vi "DIALOG_Single Element Cluster.vi"(10 "Display Items":T2[](array[typedef]), 11 "Affected Items":T1) -> (2 "Placement Out":enum32{"Choice 1", "Choice 2"}(radio), 3 "Selected Items (tags)":string[](array[string]))   [LabVIEW 2023]
uses:
  cluster/Cluster Element Description.ctl
  top/BundleMagic.ctl
panel:
  out "Cancel?":bool
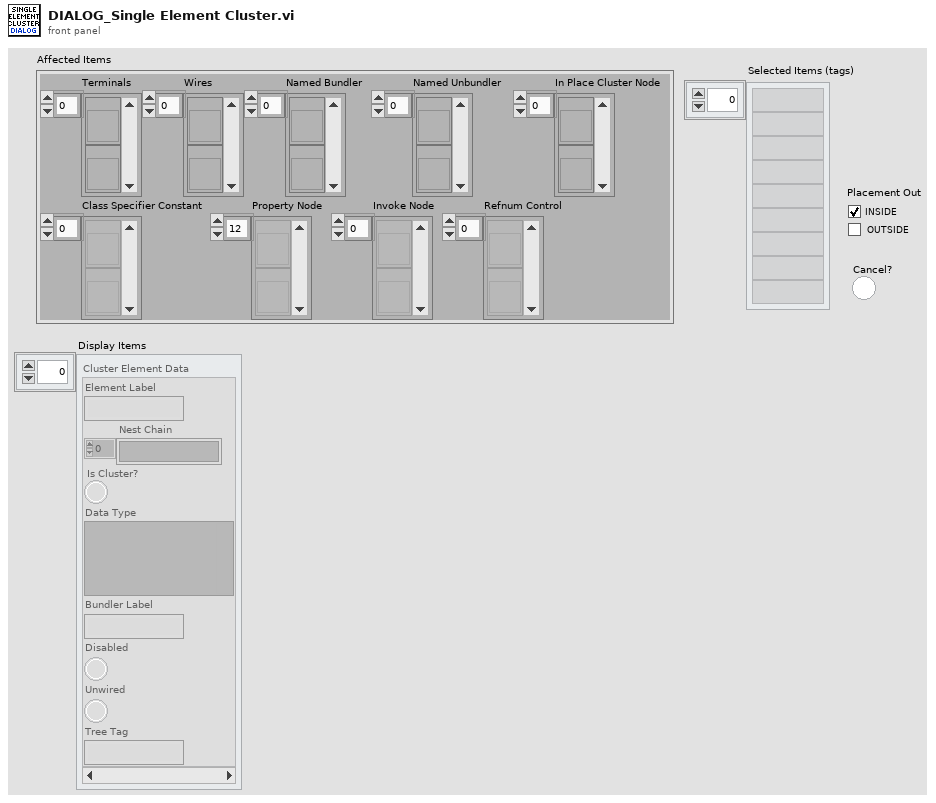
[diagram p1: front panel]
types:
  T1 = typedef "BundleMagic.ctl" = cluster{"Terminals":refnum<vi>[], "Wires":refnum<vi>[], "Named Bundler":refnum<vi>[], "Named Unbundler":refnum<vi>[], "In Place Cluster Node":refnum<vi>[], "Class Specifier Constant":refnum<vi>[], "Property Node":refnum<vi>[], "Invoke Node":refnum<vi>[], "Refnum Control":refnum<vi>[]}
  T2 = typedef "Cluster Element Description.ctl" = cluster{"Element Label":string, "Nest Chain":string[], "Is Cluster?":bool, "Data Type":variant, "Bundler Label":string, "Disabled":bool, "Unwired":bool, "Tree Tag":string}
  T3 = cluster{"Tunnel Ref":refnum<vi>, "On Tunnel?":bool, "Placement":enum32{"Choice 1", "Choice 2"}, "Tunnel Is Indexing?":bool, "Diagram":refnum<vi>, "Position":cluster{"Refnum":refnum<vi>, "Relative Direction":enum32{"Right", "Left", "Top", "Bottom", "Top Right", "Top Left", "Bottom Right", "Bottom Left"}, "Point32":cluster{"Horizontal":i32, "Vertical":i32}}, "Chosen Terminal":refnum<vi>, "Is Refnum?":bool, "Is Cluster?":bool, "Is Source?":bool, "Tunnel Direction":enum16{"In-Going", "Out-Going"}, "Tunnel Position":enum16{"Left", "Top", "Right", "Bottom"}, "Is Inner?":bool, "Terminal Is Indexing?":bool}
  T4 = enum16{"Left Button", "Center Button", "Right Button", "Window Close"}
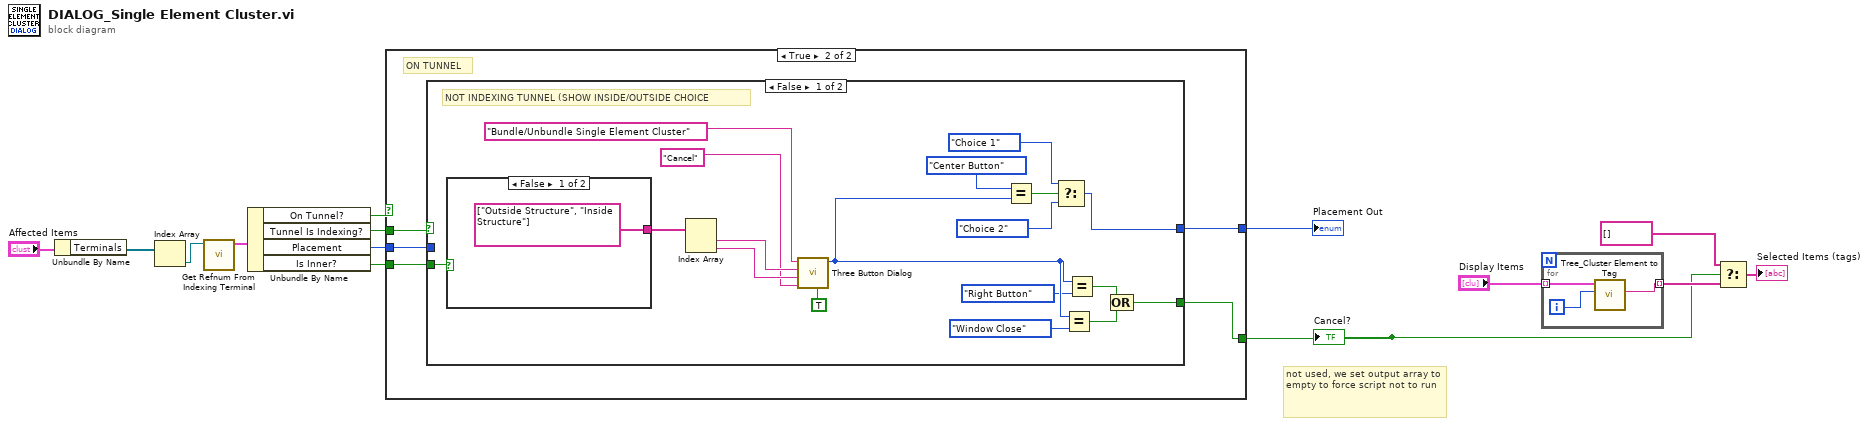
[diagram p0: block diagram]
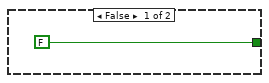
[diagram p2: hidden frame]
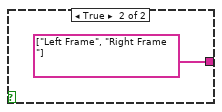
[diagram p3: hidden frame]
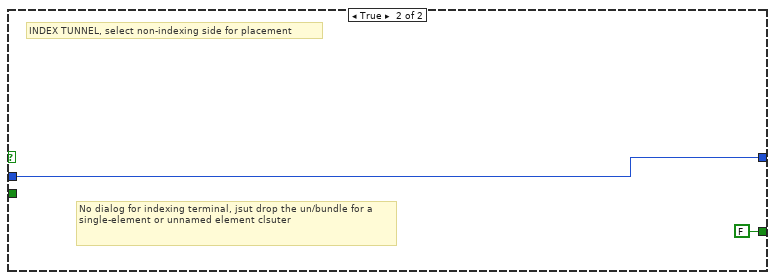
[diagram p4: hidden frame]
diagram:
  # "not used, we set output array to empty to force script not to run"
  n1 = Unbundle By Name("Affected Items") -> ("Terminals"=w13:refnum<vi>[])
  n2 = Index Array(array=w13) -> (element=w5:refnum<vi>)  [unwired: 1 in]
  n3 = call "Get Refnum From Indexing Terminal.vi"("Refnum Terminal"=w5) -> ("Terminal Data Cluster"=w6:T3)  [unwired: 8 in, 2 out]
  n4 = Unbundle By Name(w6) -> ("On Tunnel?"=w2:bool, "Tunnel Is Indexing?"=w1:bool, "Placement"=w3:enum32{"Choice 1", "Choice 2"}, "Is Inner?"=w4:bool)
  n5 = case shown="True" w2 {
    tunnel: w4 -> [_ w20]
    tunnel: [_ w18] -> w11
    tunnel: [FALSE w17] -> w8
    tunnel: w3 -> [_ w19]
    tunnel: w1 -> [_ w16]
    frame False {
    }
    frame True {
      # "ON TUNNEL"
      n6 = case shown="False" w16 {
        tunnel: w20 -> [w34 _]
        tunnel: w19 -> [_ w41]
        tunnel: [w24 w41] -> w18
        tunnel: [w23 FALSE] -> w17
        frame False {
          # "NOT INDEXING TUNNEL (SHOW INSIDE/OUTSIDE CHOICE"
          n7 = case shown="False" w34 {
            tunnel: [string[] ["Outside Structure", "Inside Structure"] string[] ["Left Frame", "Right Frame "]] -> w38
            frame False {
            }
            frame True {
            }
          }
          n8 = Index Array(array=w38) -> (element #1=w37:string, element #2=w36:string)  [unwired: 2 in]
          n9 = call <vilib>:"Three Button Dialog.vi"("Allow user to close window? (TRUE)"=TRUE, "Right Button Text (\"Cancel\")"="Cancel", "Center Button Text (\"No\")"=w36, "Left Button Text (\"Yes\")"=w37, "message"="Bundle/Unbundle Single Element Cluster") -> ("Which Button?"=w28:T4)  [unwired: 6 in]
          n10 = Equal?(x=T4."Center Button" ("Which Button?"), y=w28) -> (x = y?=w33:bool)
          n11 = Select(t=enum32{"Choice 1", "Choice 2"}."Choice 1" ("Placement Out"), s=w33, f=enum32{"Choice 1", "Choice 2"}."Choice 2" ("Placement Out")) -> (s? t:f=w24:enum32{"Choice 1", "Choice 2"})
          n12 = Equal?(x=w28, y=T4."Window Close" ("Which Button?")) -> (x = y?=w32:bool)
          n13 = Equal?(x=w28, y=T4."Right Button" ("Which Button?")) -> (x = y?=w31:bool)
          n14 = Compound Arithmetic op=OR(w31, w32) -> (w23:bool)
        }
        frame True {
          # "INDEX TUNNEL, select non-indexing side for placement"
          # "No dialog for indexing terminal, jsut drop the un/bundle for a single-element or unnamed element clsuter"
        }
      }
    }
  }
  "Placement Out" <- w11
  "Cancel?" <- w8
  n15 = for {
    tunnel: "Display Items" -> [w45] mode=indexing
    tunnel: [w43] -> w9 mode=indexing
    i -> [w44]
    n16 = call "Tree_Cluster Element to Tag.vi"("Index"=w44, "Cluster Element Data"=w45) -> ("Tree Tag Value"=w43:string)  [unwired: 8 in, 1 out]
  }
  n17 = Select(t=string[] [] ("Selected Items (tags)"), s=w8, f=w9) -> (s? t:f=→"Selected Items (tags)":string[])
